vi "LOC subGetControlFullyQualifiedLabel.vi"(4 "error in (no error)":errorcluster, 7 "reference":refnum<vi>) -> (0 "error out":errorcluster, 2 "Fully Qualified Label":string, 3 "dup reference":refnum<vi>)   [LabVIEW 2020, in "Localization_Tools.lvlib"]
uses:
  Localization_Tools.lvlib
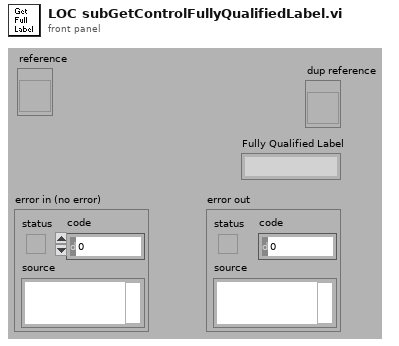
[diagram p1: front panel]
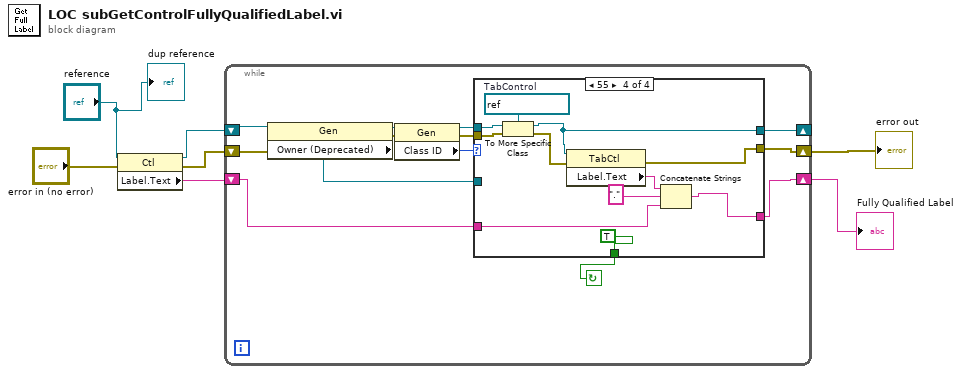
[diagram p0: block diagram]
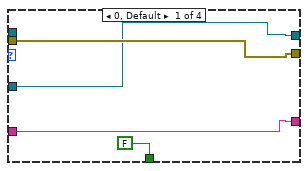
[diagram p2: hidden frame]
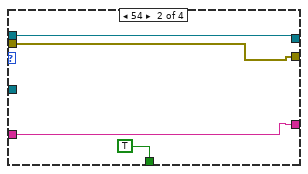
[diagram p3: hidden frame]
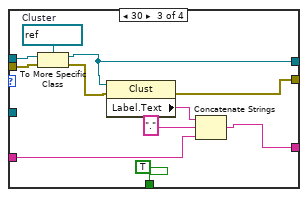
[diagram p4: hidden frame]
diagram:
  n1 = property class="Ctl"(reference="reference", error in="error in (no error)") -> (reference out=w5:refnum<vi>, error out=w6:errorcluster, "Label.Text"=w7:string)
  n2 = while {
    shift-right: [w15] -> _
    shift-left: w5 -> [w17]
    shift-right: [w14] -> w2
    shift-left: w7 -> [w16]
    shift-right: [w11] -> w4
    shift-left: w6 -> [w12]
    stop <- w8 continue-if-true
    n3 = property class="Gen"(reference=w17, error in=w12) -> (error out=w10:errorcluster, "Owner (Deprecated)"=w19:refnum<vi>)  [unwired: 1 out]
    n4 = property class="Gen"(reference=w19, error in=w10) -> (reference out=w18:refnum<vi>, error out=w13:errorcluster, "Class ID"=w9:u32)
    n5 = case shown="55" w9 {
      tunnel: w18 -> [_ w24 w38 w49]
      tunnel: w17 -> [w22 _ _ _]
      tunnel: w16 -> [w21 w26 w36 w47]
      tunnel: [w22 w24 w30 w41] -> w15
      tunnel: [w21 w26 w31 w42] -> w14
      tunnel: w13 -> [w23 w27 w33 w44]
      tunnel: [w23 w27 w32 w43] -> w11
      tunnel: [FALSE TRUE TRUE TRUE] -> w8
      frame 0, Default {
      }
      frame 54 {
      }
      frame 30 {
        w37 = refnum<vi> refnum  # Cluster
        n6 = To More Specific Class(target class=w37, reference=w38, error in=w33) -> (specific class reference=w30:refnum<vi>, error out=w29:errorcluster)
        n7 = property class="Clust"(reference=w30, error in=w29) -> (error out=w32:errorcluster, "Label.Text"=w34:string)  [unwired: 1 out]
        n8 = Concatenate Strings(w34, ".", w36) -> (w31:string)
      }
      frame 55 {
        w48 = refnum<vi> refnum  # TabControl
        n9 = To More Specific Class(target class=w48, reference=w49, error in=w44) -> (specific class reference=w41:refnum<vi>, error out=w40:errorcluster)
        n10 = property class="TabCtl"(reference=w41, error in=w40) -> (error out=w43:errorcluster, "Label.Text"=w45:string)  [unwired: 1 out]
        n11 = Concatenate Strings(w45, ".", w47) -> (w42:string)
      }
    }
  }
  "error out" <- w4
  "Fully Qualified Label" <- w2
  "dup reference" <- "reference"
